vi "RESP3 Parser Example.vi"() -> ()   [LabVIEW 2019]
uses:
  RESP3/RESP3 Parser/RESP3 Parser.lvclass
  RESP3/high-level/RESP3 Get Array.vi
  RESP3/high-level/RESP3 Get Double.vi
  RESP3/high-level/RESP3 Get String.vi
  RESP3/RESP3.lvlib
panel:
  out "second element":dbl
  out "first element":string
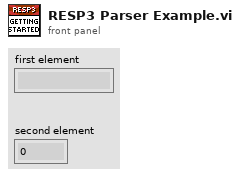
[diagram p1: front panel]
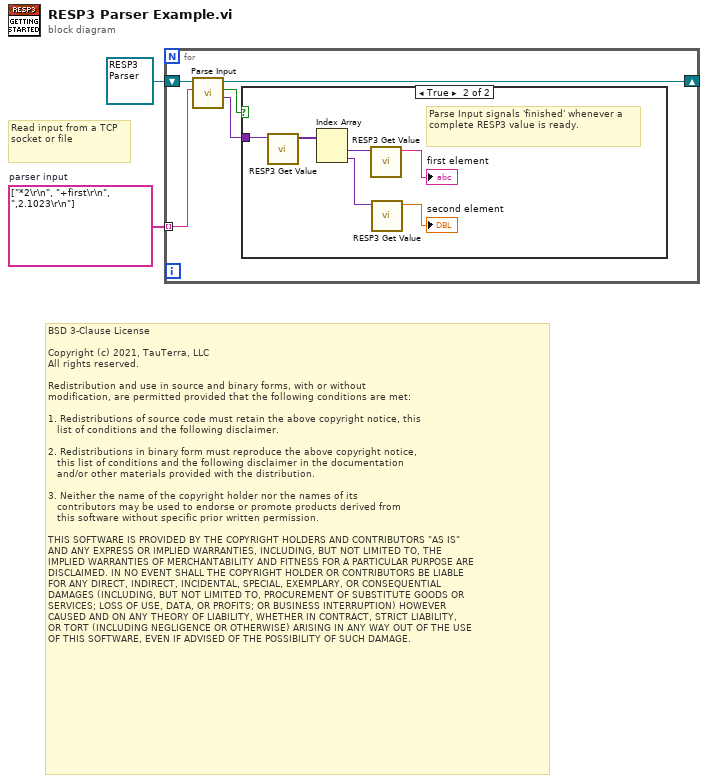
[diagram p0: block diagram]
diagram:
  w1 = string[] ["*2\r\n", "+first\r\n", ",2.1023\r\n"]  # parser input
  # "BSD 3-Clause License\n\nCopyright (c) 2021, TauTerra, LLC\nAll rights reserved.\n\nRedistribution and use in source and binary forms, with or without\nmodification, are permitted provided that the following conditions are met:\n\n1. Redistributions of source code must retain the above copyright notice, this\n   list of conditions and the following disclaimer.\n\n2. Redistributions in binary form must reproduce the above copyright notice,\n   this list of conditions and the following disclaimer in the documentation\n   and/or other materials provided with the distribution.\n\n3. Neither the name of the copyright holder nor the names of its\n   contributors may be used to endorse or promote products derived from\n   this software without specific prior written permission.\n\nTHIS SOFTWARE IS PROVIDED BY THE COPYRIGHT HOLDERS AND CONTRIBUTORS \"AS IS\"\nAND ANY EXPRESS OR IMPLIED WARRANTIES, INCLUDING, BUT NOT LIMITED TO, THE\nIMPLIED WARRANTIES OF MERCHANTABILITY AND FITNESS FOR A PARTICULAR PURPOSE ARE\nDISCLAIMED. IN NO EVENT SHALL THE COPYRIGHT HOLDER OR CONTRIBUTORS BE LIABLE\nFOR ANY DIRECT, INDIRECT, INCIDENTAL, SPECIAL, EXEMPLARY, OR CONSEQUENTIAL\nDAMAGES (INCLUDING, BUT NOT LIMITED TO, PROCUREMENT OF SUBSTITUTE GOODS OR\nSERVICES; LOSS OF USE, DATA, OR PROFITS; OR BUSINESS INTERRUPTION) HOWEVER\nCAUSED AND ON ANY THEORY OF LIABILITY, WHETHER IN CONTRACT, STRICT LIABILITY,\nOR TORT (INCLUDING NEGLIGENCE OR OTHERWISE) ARISING IN ANY WAY OUT OF THE USE\nOF THIS SOFTWARE, EVEN IF ADVISED OF THE POSSIBILITY OF SUCH DAMAGE."
  # "Read input from a TCP socket or file"
  n1 = for {
    shift-right: [w6] -> _
    shift-left: refnum<class "RESP3 Parser.lvclass"> refnum ("RESP3.lvlib:RESP3 Parser.lvclass") -> [w7]
    tunnel: w1 -> [w5] mode=indexing
    n2 = call-dynamic "Parse Input.vi"("input line"=w5, "RESP3 Parser in"=w7) -> ("RESP3 Value"=w3:variant, "finished?"=w4:bool, "RESP3 Parser out"=w6:refnum<class "RESP3 Parser.lvclass">)  [unwired: 5 in, 2 out]
    n3 = case shown="True" w4 {
      tunnel: w3 -> [_ w13]
      frame False {
      }
      frame True {
        # "Parse Input signals 'finished' whenever a complete RESP3 value is ready."
        n4 = call-poly "RESP3 Get Value.vi"("RESP3 Value in"=w13) -> ("RESP3 Values out"=w12:variant[])  [unwired: 7 in, 3 out]
        n5 = Index Array(array=w12) -> (element #1=w11:variant, element #2=w10:variant)  [unwired: 2 in]
        n6 = call-poly "RESP3 Get Value.vi"("RESP3 Value in"=w11) -> ("String out"=→"first element":string)  [unwired: 7 in, 3 out]
        n7 = call-poly "RESP3 Get Value.vi"("RESP3 Value in"=w10) -> ("Number out"=→"second element":dbl)  [unwired: 8 in, 2 out]
      }
    }
  }
